vi "rms_minus_dc.vi"(10 "Signal":T1) -> (2 "RMS":dbl[](array[numeric]), 3 "DC":dbl[](array[numeric]), 4 "AC signal":waveform(sgl)[](array[waveform]))   [LabVIEW 2011]
panel:
  # "3D RMS in last element"
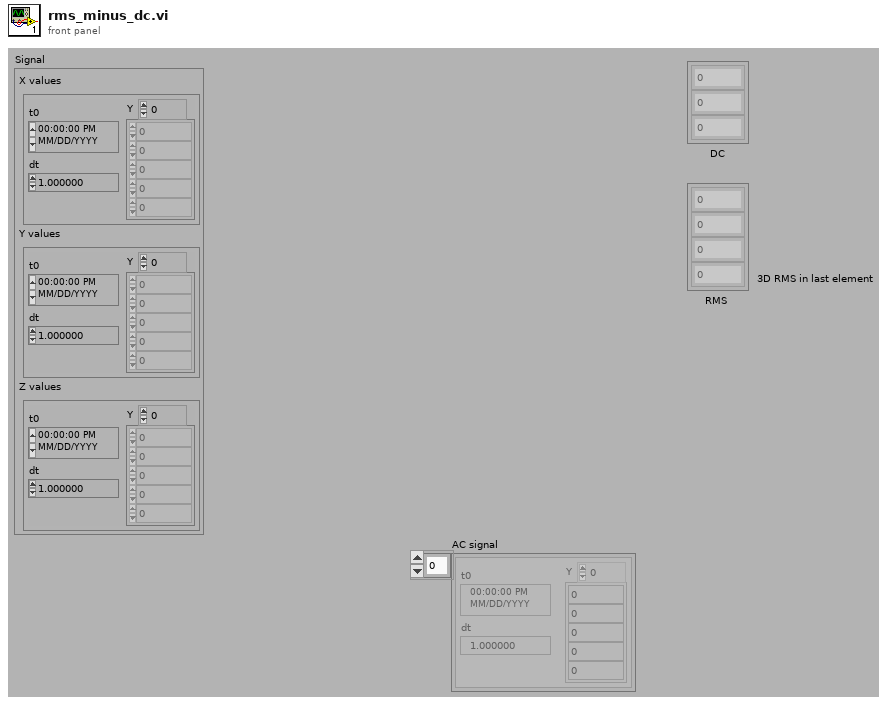
[diagram p1: front panel]
types:
  T1 = cluster{"X values":waveform(sgl), "Y values":waveform(sgl), "Z values":waveform(sgl)}
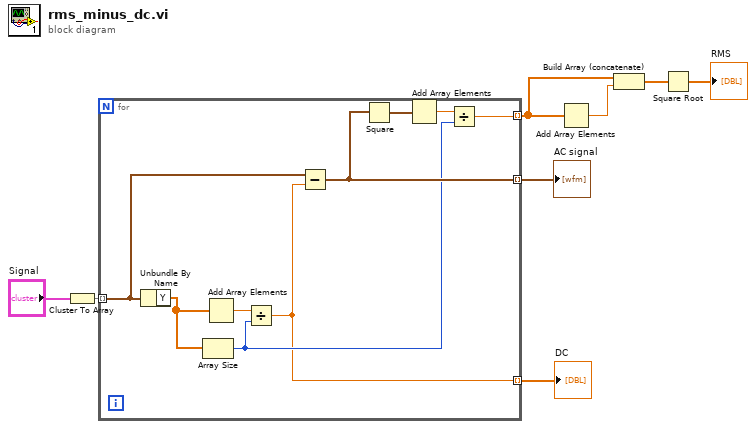
[diagram p0: block diagram]
diagram:
  n1 = Cluster To Array(cluster="Signal") -> (array=w7:waveform(sgl)[])
  n2 = for {
    tunnel: w7 -> [w16] mode=indexing
    tunnel: [w15] -> w5 mode=indexing
    tunnel: [w11] -> w6 mode=indexing
    tunnel: [w10] -> w3 mode=indexing
    n3 = Unbundle By Name(w16) -> ("Y"=w9:sgl[])
    n4 = Array Size(array=w9) -> (size(s)=w12:i32)
    n5 = Add Array Elements(numeric array=w9) -> (sum=w17:sgl)
    n6 = Divide(x=w17, y=w12) -> (x/y=w11:sgl)
    n7 = Subtract(x=w16, y=w11) -> (x-y=w15:waveform(sgl))
    n8 = Square(x=w15) -> (x^2=w14:waveform(sgl))
    n9 = Add Array Elements(numeric array=w14) -> (sum=w13:sgl)
    n10 = Divide(x=w13, y=w12) -> (x/y=w10:sgl)
  }
  "DC" <- w6
  "AC signal" <- w5
  n11 = Add Array Elements(numeric array=w3) -> (sum=w4:sgl)
  n12 = Build Array (concatenate)(w3, w4) -> (w2:sgl[])
  n13 = Square Root(x=w2) -> (sqrt(x)=→"RMS":sgl[])
